vi "Line_distance.vi"(9 "Num. of Drops in":dbl, 10 "Pitch in":dbl[](array[numeric]), 11 "Dist. b/w Lines in":dbl[](array[numeric])) -> (3 "Array":dbl[](array[numeric]))   [LabVIEW 2021]
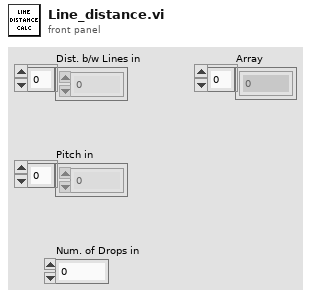
[diagram p1: front panel]
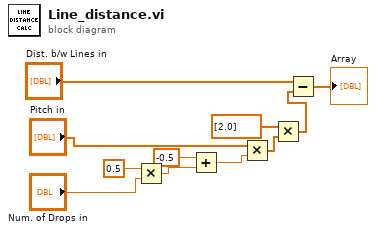
[diagram p0: block diagram]
diagram:
  n1 = Multiply(x=0.5, y="Num. of Drops in") -> (x*y=w6:dbl)
  n2 = Add(x=-0.5, y=w6) -> (x+y=w7:dbl)
  n3 = Multiply(x="Pitch in", y=w7) -> (x*y=w2:dbl[])
  n4 = Multiply(x=dbl[] [2.0], y=w2) -> (x*y=w3:dbl[])
  n5 = Subtract(x="Dist. b/w Lines in", y=w3) -> (x-y=→"Array":dbl[])
